vi "Read Value.vi"(7 "AnalogIn":refnum<class "AnalogIn.lvclass">, 8 "error in (no error)":errorcluster, 11 "Session In":refnum<class "Session.lvclass">) -> (0 "error out":errorcluster, 2 "Value":T1, 3 "Session Out":refnum<class "Session.lvclass">)   [LabVIEW 2020, in "CTI.lvlib" / "AnalogIn.lvclass"]
uses:
  AnalogIn.lvclass
  Session/Session.lvclass
  Raw ADC.ctl
  CTI.lvlib
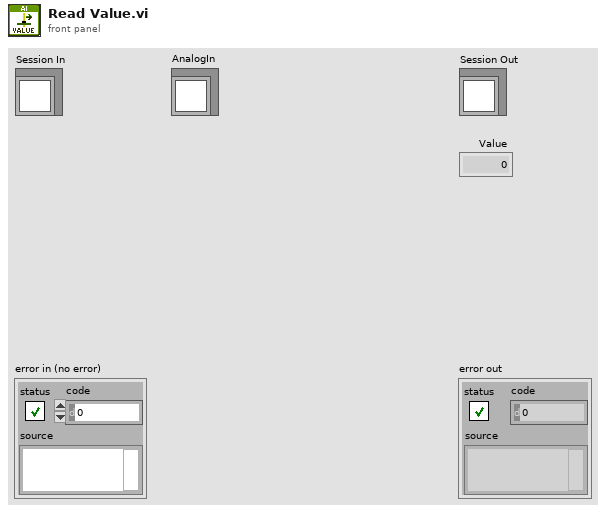
[diagram p1: front panel]
types:
  T1 = typedef "CTI.lvlib/Raw ADC.ctl" = u16
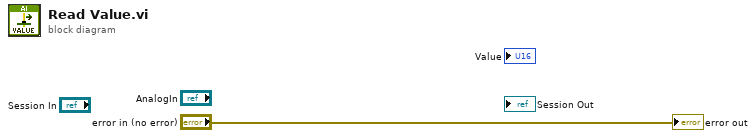
[diagram p0: block diagram]
diagram:
  "error out" <- "error in (no error)"
